vi "Get Frame Position (Time).vi"(8 "error in (no error)":errorcluster, 11 "Reader in":refnum<class "Reader.lvclass">) -> (0 "error out":errorcluster, 2 "Time (ms)":u64, 3 "Reader":refnum<class "Reader.lvclass">)   [LabVIEW 2020, in "video_io.lvlib" / "Reader.lvclass"]
uses:
  Reader.lvclass
  Reader.lvclass/Reader.ctl
  acb2feee-aaa4-4f40-955f-c8ac8e9dff35.vi
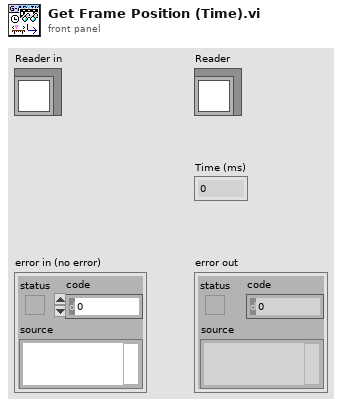
[diagram p1: front panel]
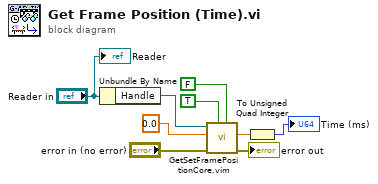
[diagram p0: block diagram]
diagram:
  n1 = Unbundle By Name("Reader in") -> ("Handle"=w9:refnum<data-value>)
  n2 = call "GetSetFramePositionCore.vim"("As Frame Index"=FALSE ("Get"), "Get"=TRUE, "error in (no error)"="error in (no error)", "Position In"=0.0, "Handle"=w9) -> ("error out"=→"error out":errorcluster, "Position Out"=w2:dbl)  [unwired: 5 in]
  n3 = To Unsigned Quad Integer(1:w2) -> (0:→"Time (ms)":u64)
  "Reader" <- "Reader in"
